vi "Find Test Cases in LVProj.vi"(8 "error in (no error)":errorcluster, 11 "Project Path":path) -> (0 "error out":errorcluster, 2 "Class paths":path[](array[path]), 3 "Classes in project":string[](array[string]))   [LabVIEW 2020, in "Test Finder.lvclass"]
uses:
  Test Finder.lvclass
  Utilities/Utilities.lvlib
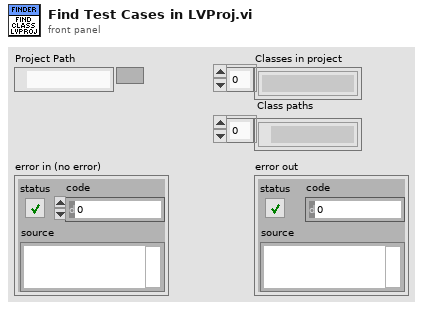
[diagram p1: front panel]
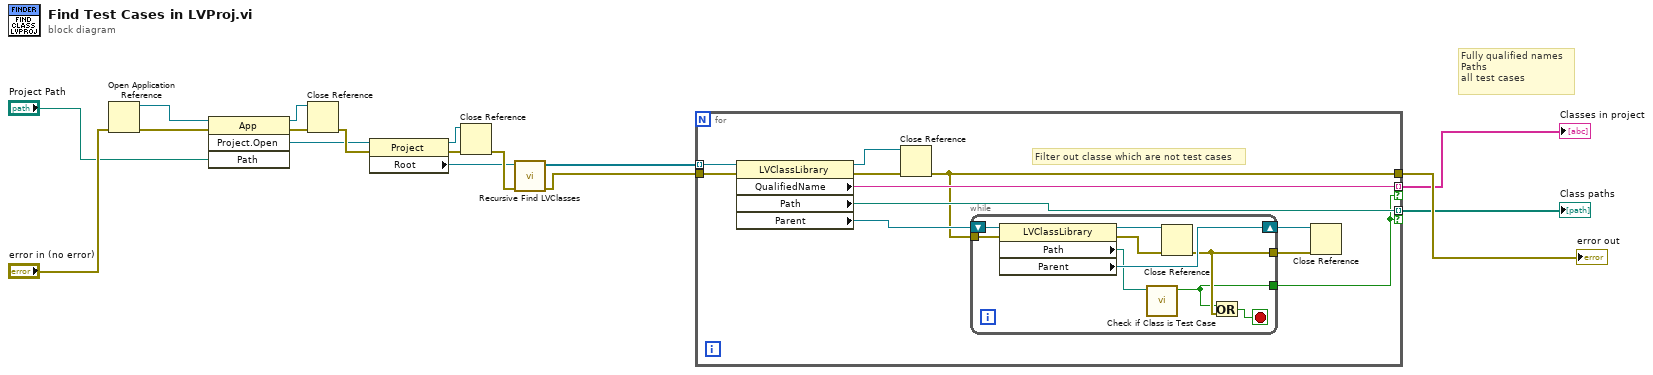
[diagram p0: block diagram]
diagram:
  # "Fully qualified names\nPaths\nall test cases"
  n1 = Open Application Reference(8:"error in (no error)") -> (0:w6:errorcluster, 3:w5:refnum<vi>)  [unwired: 3 in]
  n2 = invoke class="App" method="Project.Open"(reference=w5, error in=w6, "Path"="Project Path") -> (reference out=w8:refnum<vi>, error out=w7:errorcluster, "Project:Open"=w9:refnum<vi>)  [unwired: 1 in, 1 out]
  n3 = Close Reference(reference=w8, error in (no error)=w7) -> (error out=w10:errorcluster)
  n4 = property class="Project"(reference=w9, error in=w10) -> (reference out=w17:refnum<vi>, error out=w11:errorcluster, "Root"=w1:refnum<vi>)
  n5 = Close Reference(reference=w17, error in (no error)=w11) -> (error out=w16:errorcluster)
  n6 = call "Recursive Find LVClasses.vi"("error in (no error)"=w16, "reference"=w1) -> ("error out"=w2:errorcluster, "Class References"=w12:refnum<vi>[])  [unwired: 8 in]
  n7 = for {
    tunnel: w12 -> [w28] mode=indexing
    tunnel: w2 -> [w27]
    tunnel: [w26] -> w13 mode=indexing if=w21
    tunnel: [w20] -> w15
    tunnel: [w25] -> w3 mode=indexing if=w21
    # "Filter out classe which are not test cases"
    n8 = property class="LVClassLibrary"(reference=w28, error in=w27) -> (reference out=w23:refnum<vi>, error out=w24:errorcluster, "QualifiedName"=w26:string, "Path"=w25:path, "Parent"=w22:refnum<vi>)
    n9 = Close Reference(reference=w23, error in (no error)=w24) -> (error out=w20:errorcluster)
    n10 = while {
      tunnel: w20 -> [w36]
      tunnel: [w29] -> w21
      shift-right: [w32] -> w19
      shift-left: w22 -> [w37]
      tunnel: [w31] -> w18
      stop <- w33 stop-if-true
      n11 = property class="LVClassLibrary"(reference=w37, error in=w36) -> (reference out=w34:refnum<vi>, error out=w35:errorcluster, "Path"=w30:path, "Parent"=w32:refnum<vi>)
      n12 = call "Check if Class is Test Case.vi"("Path"=w30) -> ("Is Test Case?"=w29:bool)  [unwired: 9 in, 1 out]
      n13 = Close Reference(reference=w34, error in (no error)=w35) -> (error out=w31:errorcluster)
      n14 = Or(x=w29, y=w31) -> (x .or. y?=w33:bool)
    }
    n15 = Close Reference(reference=w19, error in (no error)=w18) -> ()  [unwired: 1 out]
  }
  "error out" <- w15
  "Classes in project" <- w13
  "Class paths" <- w3
